vi "Conductus Load Calibration.vi"(4 "Error In":errorcluster, 5 "Voltage Bias":T1(ring)=enum."3 mV", 6 "Sensor Type":T2(ring)=enum."Resistance1.0M ", 7 "Instrument Address":refnum<visa-resource-name>) -> (0 "error out":errorcluster, 3 "dup VISA session":refnum<visa-resource-name>)   [LabVIEW 2021]
doc: "This VI loads a calibration file into the Conductus LTC-20 temperature controller. The file is a line of up to 19 characters of ID info, followed by the temperature information in 2 columns of temperature and resistance (sensor value)\nScott Hannahs, NHMFL-FSU, March 1995"
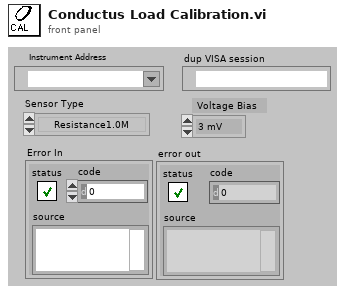
[diagram p1: front panel]
types:
  T1 = enum16{"10 mV", "3 mV", "1 mV", "320 uV", "100 uV", "32 uV", "10 uV"}
  T2 = enum16{"2V Diode", "6V Diode", "Platinum - 1 mA", "Platinum - 100µA", "Resistance1.0M "}
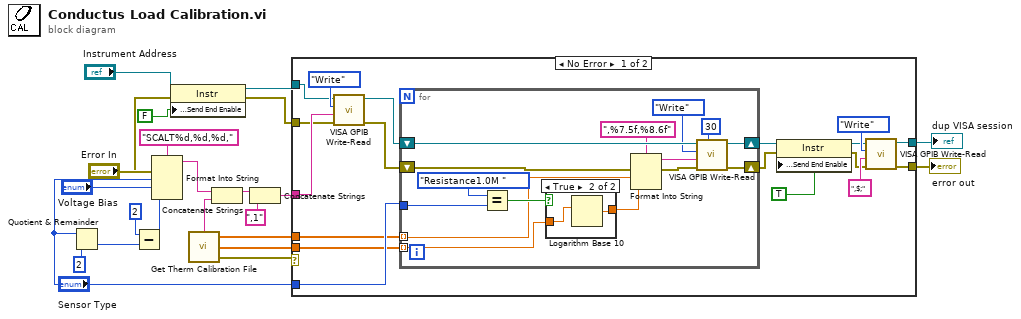
[diagram p0: block diagram]
diagram:
  n1 = Quotient & Remainder(x="Sensor Type", y=2) -> (floor(x/y)=w22:i32)  [unwired: 1 out]
  n2 = Subtract(x=2, y=w22) -> (x-y=w19:i32)
  n3 = Format Into String(format string="SCALT%d,%d,%d," ("Format String"), error in="Error In", "Sensor Type", "Voltage Bias", w19) -> (resulting string=w7:string, error out=w2:errorcluster)  [unwired: 1 in]
  n4 = property class="Instr"(reference="Instrument Address", error in=w2, "Message Based Settings:Send End Enable"=FALSE) -> (reference out=w5:refnum<visa-resource-name>, error out=w3:errorcluster)
  n5 = call "Get Therm Calibration File.vi"() -> ("Calbration Name"=w8:string, "Temperature"=w12:dbl[], "Resistance"=w11:dbl[], "error out"=w13:errorcluster)  [unwired: 1 in]
  n6 = Concatenate Strings(w7, w8) -> (w9:string)
  n7 = Concatenate Strings(w9, ",1") -> (w6:string)
  n8 = case shown="No Error" w13 {
    tunnel: w6 -> [w37 _]
    tunnel: "Sensor Type" -> [w41 _]
    tunnel: [w32 w61] -> w15
    tunnel: w3 -> [w36 w61]
    tunnel: w5 -> [w38 w60]
    tunnel: [w31 w60] -> w14
    tunnel: w12 -> [w30 _]
    tunnel: w11 -> [w29 _]
    frame No Error {
      n9 = call "VISA GPIB Write-Read.vi"("error in (no error)"=w36, "Command"=w37, "Action"=enum16{"Write", "Read", "Write & Read"}."Write", "VISA resource name"=w38) -> ("error out"=w35:errorcluster, "dup VISA Session"=w33:refnum<visa-resource-name>)  [unwired: 4 in, 2 out]
      n10 = for {
        tunnel: w41 -> [w56]
        shift-right: [w51] -> w27
        shift-left: w35 -> [w53]
        shift-right: [w52] -> w28
        shift-left: w33 -> [w50]
        tunnel: w30 -> [w49] mode=indexing
        tunnel: w29 -> [w42] mode=indexing
        n11 = Equal?(x=T2."Resistance1.0M ", y=w56) -> (x = y?=w55:bool)
        n12 = case shown="True" w55 {
          tunnel: w42 -> [w57 w59]
          tunnel: [w57 w58] -> w43
          frame False {
          }
          frame True {
            n13 = Logarithm Base 10(1:w59) -> (0:w58:dbl)
          }
        }
        n14 = Format Into String(format string=",%7.5f,%8.6f" ("Format String"), error in=w53, w49, w43) -> (resulting string=w46:string, error out=w44:errorcluster)  [unwired: 1 in]
        n15 = call "VISA GPIB Write-Read.vi"("Wait (ms)"=u32 30 ("wait (mS)"), "error in (no error)"=w44, "Command"=w46, "Action"=enum16{"Write", "Read", "Write & Read"}."Write", "VISA resource name"=w50) -> ("error out"=w51:errorcluster, "dup VISA Session"=w52:refnum<visa-resource-name>)  [unwired: 3 in, 2 out]
      }
      n16 = property class="Instr"(reference=w28, error in=w27, "Message Based Settings:Send End Enable"=TRUE) -> (reference out=w25:refnum<visa-resource-name>, error out=w24:errorcluster)
      n17 = call "VISA GPIB Write-Read.vi"("error in (no error)"=w24, "Command"=",$;", "Action"=enum16{"Write", "Read", "Write & Read"}."Write", "VISA resource name"=w25) -> ("error out"=w32:errorcluster, "dup VISA Session"=w31:refnum<visa-resource-name>)  [unwired: 4 in, 2 out]
    }
    frame Error {
    }
  }
  "dup VISA session" <- w14
  "error out" <- w15
